vi "IC_FlipFilter.vi"(0 "ICImagingControl":refnum<k7>, 1 "Top":i32, 2 "Left":i32, 3 "Height":i32, 4 "Width":i32) -> (5 "ICImagingControl 2":refnum<k7>, 6 "ROI":refnum<k7>)   [LabVIEW 2020]
doc: "This VI inserts an ROI frame filter in the device path of IC Imaging Control."
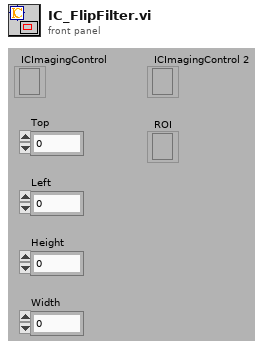
[diagram p1: front panel]
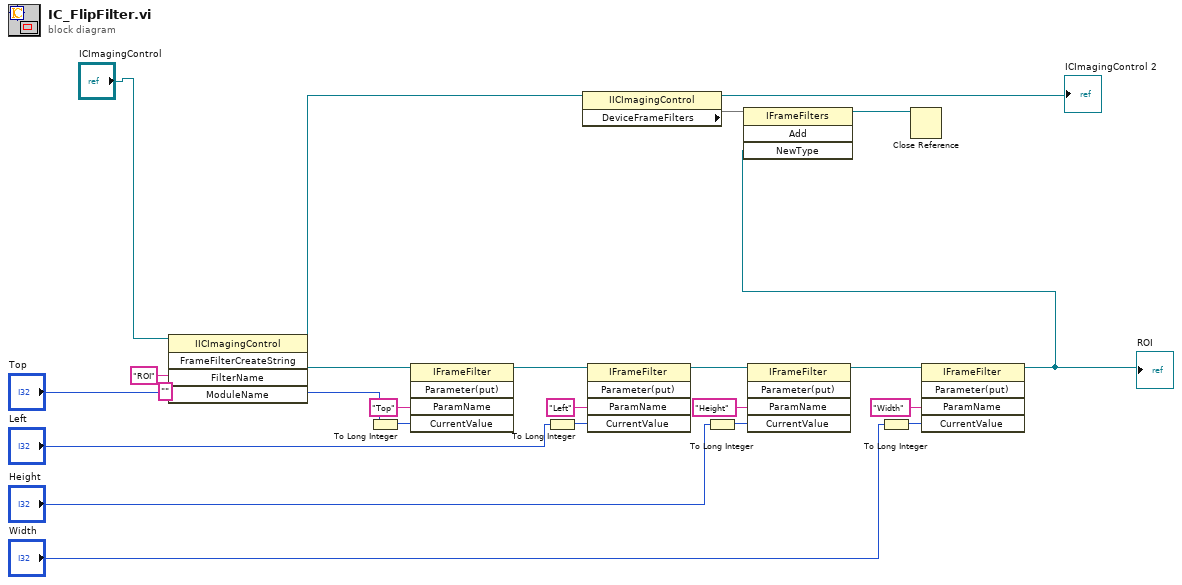
[diagram p0: block diagram]
diagram:
  n1 = invoke class="IICImagingControl" method="FrameFilterCreateString"(reference="ICImagingControl", "FilterName"="ROI", "ModuleName"="") -> (reference out=w5:refnum<k7>, "FrameFilterCreateString"=w8:refnum<k7>)  [unwired: 2 in, 3 out]
  n2 = To Long Integer(number="Top") -> (32bit integer=w10:i32)
  n3 = invoke class="IFrameFilter" method="Parameter(put)"(reference=w8, "ParamName"="Top", "CurrentValue"=w10) -> (reference out=w14:refnum<k7>)  [unwired: 2 in, 4 out]
  n4 = To Long Integer(number="Left") -> (32bit integer=w13:i32)
  n5 = property class="IICImagingControl"(reference=w5) -> (reference out=→"ICImagingControl 2":refnum<k7>, "DeviceFrameFilters"=w4)  [unwired: 1 in, 1 out]
  n6 = invoke class="IFrameFilter" method="Parameter(put)"(reference=w14, "ParamName"="Left", "CurrentValue"=w13) -> (reference out=w18:refnum<k7>)  [unwired: 2 in, 4 out]
  n7 = To Long Integer(number="Height") -> (32bit integer=w17:i32)
  n8 = invoke class="IFrameFilter" method="Parameter(put)"(reference=w18, "ParamName"="Height", "CurrentValue"=w17) -> (reference out=w21:refnum<k7>)  [unwired: 2 in, 4 out]
  n9 = To Long Integer(number="Width") -> (32bit integer=w20:i32)
  n10 = invoke class="IFrameFilter" method="Parameter(put)"(reference=w21, "ParamName"="Width", "CurrentValue"=w20) -> (reference out=w3:refnum<k7>)  [unwired: 2 in, 4 out]
  "ROI" <- w3
  n11 = invoke class="IFrameFilters" method="Add"(reference=w4, "NewType"=w3) -> (reference out=w1:refnum<k7>)  [unwired: 2 in, 3 out]
  n12 = Close Reference(reference=w1) -> ()  [unwired: 1 in, 1 out]
